vi "Copy Template Files.vi"(8 "error in (no error)":errorcluster, 11 "Base Path":path) -> (0 "error out":errorcluster)   [LabVIEW 2027]
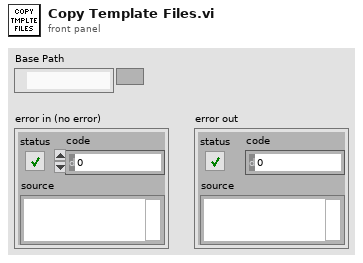
[diagram p1: front panel]
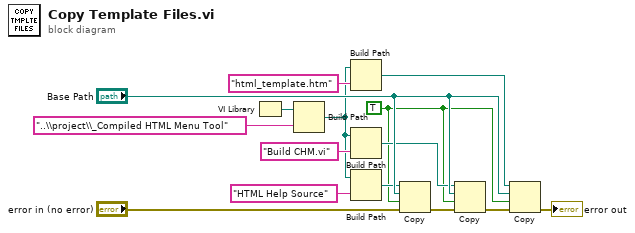
[diagram p0: block diagram]
diagram:
  w4 = TRUE ("overwrite (F)")
  n1 = VI Library() -> (path=w3:path)
  n2 = Build Path(base path=w3, name or relative path="..\\project\\_Compiled HTML Menu Tool") -> (appended path=w1:path)
  n3 = Build Path(base path=w1, name or relative path="html_template.htm") -> (appended path=w12:path)
  n4 = Build Path(base path=w1, name or relative path="Build CHM.vi") -> (appended path=w9:path)
  n5 = Build Path(base path=w1, name or relative path="HTML Help Source") -> (appended path=w6:path)
  n6 = Copy(8:"error in (no error)", 9:w4, 10:"Base Path", 11:w6) -> (0:w10:errorcluster)  [unwired: 1 in, 2 out]
  n7 = Copy(8:w10, 9:w4, 10:"Base Path", 11:w9) -> (0:w13:errorcluster)  [unwired: 1 in, 2 out]
  n8 = Copy(8:w13, 9:w4, 10:"Base Path", 11:w12) -> (0:→"error out":errorcluster)  [unwired: 1 in, 2 out]
